vi "RichToFlatcif_plugincore_MonitorI64.vi"(5 "OutputClusterType":T1, 11 "InputCluster":T2) -> (3 "OutputCluster":T1)   [LabVIEW 2021, in "CIFCorePlugin_server.lvlib"]
uses:
  CIFCorePlugin_server.lvlib
  cif_plugincore_MonitorI64.ctl
  cif_plugincore_MonitorI64_Flat.ctl
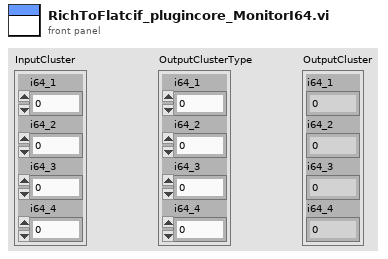
[diagram p1: front panel]
types:
  T1 = typedef "CIFCorePlugin_server.lvlib/cif_plugincore_MonitorI64_Flat.ctl" = cluster{"i64_1":i64, "i64_2":i64, "i64_3":i64, "i64_4":i64}
  T2 = typedef "CIFCorePlugin_server.lvlib/cif_plugincore_MonitorI64.ctl" = cluster{"i64_1":i64, "i64_2":i64, "i64_3":i64, "i64_4":i64}
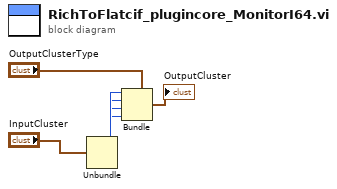
[diagram p0: block diagram]
diagram:
  n1 = Unbundle "Unbundle"("InputCluster") -> ("i64_1"=w4:i64, "i64_2"=w3:i64, "i64_3"=w2:i64, "i64_4"=w1:i64)
  n2 = Bundle "Bundle"(cluster="OutputClusterType", "i64_1"=w4, "i64_2"=w3, "i64_3"=w2, "i64_4"=w1) -> (→"OutputCluster":T1)
